vi "TM-620 Sensor Reading.vi"(3 "error in (no error)":errorcluster, 4 "channel":enum16{"Chan A", "Chan B", "Chan C", "Chan D"}(ring), 5 "VISA session":refnum<visa-resource-name>) -> (0 "error out":errorcluster, 1 "response out":string, 2 "dup VISA session":refnum<visa-resource-name>)   [LabVIEW 2019]
doc: "TM-600 Sensor Reading.vi will return the present sensor reading for a specified channel. A new reading is not initiated."
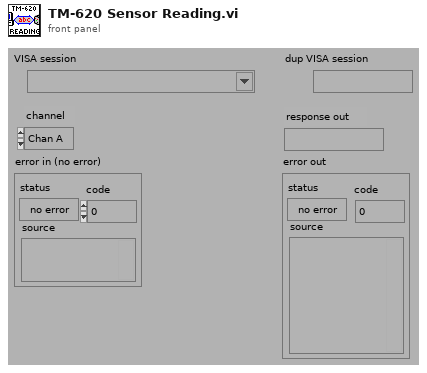
[diagram p1: front panel]
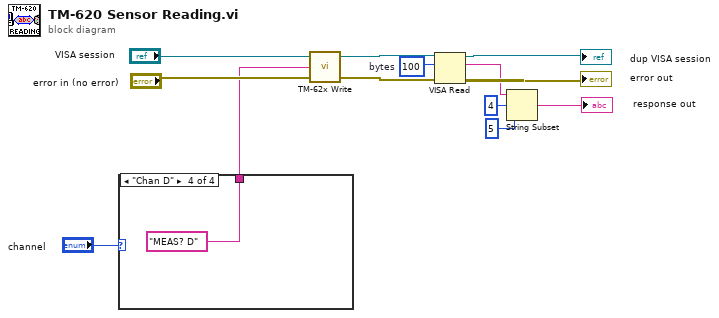
[diagram p0: block diagram]
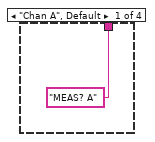
[diagram p2: hidden frame]
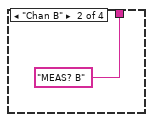
[diagram p3: hidden frame]
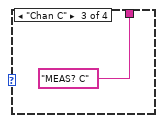
[diagram p4: hidden frame]
diagram:
  w8 = u32 100  # bytes
  n1 = case shown="\"Chan D\"" "channel" {
    tunnel: ["MEAS? A" "MEAS? B" "MEAS? C" "MEAS? D"] -> w5
    frame "Chan A", Default {
    }
    frame "Chan B" {
    }
    frame "Chan C" {
    }
    frame "Chan D" {
    }
  }
  n2 = call "TM-62x Write.vi"("error in (no error)"="error in (no error)", "write buffer (\"\")"=w5, "VISA session"="VISA session") -> ("error out"=w10:errorcluster, "dup VISA session"=w11:refnum<visa-resource-name>)  [unwired: 1 out]
  n3 = VISA Read(VISA resource name=w11, byte count=w8, error in (no error)=w10) -> (VISA resource name out=→"dup VISA session":refnum<visa-resource-name>, read buffer=w3:string, error out=→"error out":errorcluster)  [unwired: 1 out]
  n4 = String Subset(string=w3, offset (0)=4, length (rest)=5 ("length (rest)")) -> (substring=→"response out":string)
